vi "Create Error.vi"(7 "source vi name":string, 11 "error":T1=enum."Out of Bounds") -> (1 "new offset":i32, 3 "error out":errorcluster)   [LabVIEW 2016, in "Memory Manager.lvlib" / "Pointer.lvclass"]
uses:
  Pointer.lvclass
  Errors.ctl
  Constants/Library Name.vi
  VIs/New Error Cluster Constant (512B).vi
  Static Error Handling.lvlib
  Memory Manager.lvlib
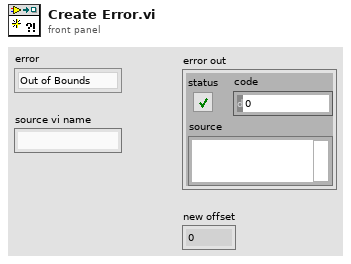
[diagram p1: front panel]
types:
  T1 = typedef "Memory Manager.lvlib/Pointer.lvclass/Errors.ctl" = enum16{"No Error", "Null Pointer", "Out of Bounds", "Buffer Underflow", "Size Mismatch", "Zone"}
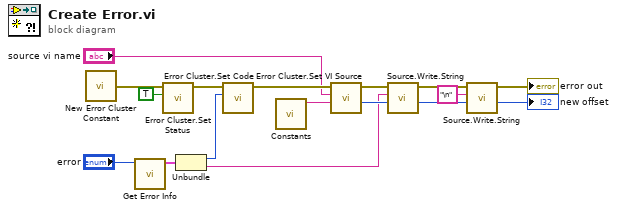
[diagram p0: block diagram]
diagram:
  n1 = call-poly "New Error Cluster Constant.vi"() -> ("error out"=w1:errorcluster)  [unwired: 1 in]
  n2 = call "Get Error Info.vi"("error"="error") -> ("error info"=w12:cluster{"code":i32, "description":string})  [unwired: 10 in]
  n3 = call "Error Cluster.Set Status.vi"("status (T)"=TRUE, "error in"=w1) -> ("error out"=w15:errorcluster)  [unwired: 9 in]
  n4 = Unbundle(w12) -> ("code"=w10:i32, "description"=w7:string)
  n5 = call "Error Cluster.Set Code.vi"("code"=w10, "error in"=w15) -> ("error out"=w16:errorcluster)  [unwired: 9 in]
  n6 = call-poly "Constants.vi"() -> ("library name"=w17:string)  [unwired: 11 in]
  n7 = call "Error Cluster.Set VI Source.vi"("library name (\"\")"=w17, "vi name"="source vi name", "error in"=w16) -> ("new offset"=w8:i32, "error out"=w9:errorcluster)  [unwired: 7 in]
  n8 = call "Source.Write.String.vi"("offset"=w8, "string"=w7, "error in"=w9) -> ("new offset"=w4:i32, "error out"=w6:errorcluster)  [unwired: 7 in]
  n9 = call "Source.Write.String.vi"("offset"=w4, "string"="\n", "error in"=w6) -> ("new offset"=→"new offset":i32, "error out"=→"error out":errorcluster)  [unwired: 7 in]
